vi "viscosity_to_RPM_derate.vi"(8 "base RPM":dbl=350.0, 9 "slope":dbl=-5.2, 10 "viscosity (cP)":dbl) -> (3 "output_RPM":i32)   [LabVIEW 2019]
panel:
  out "output_base_RPM":dbl=380.0
  in  "min_RPM":i32=30
  out "desired_RPM":i32
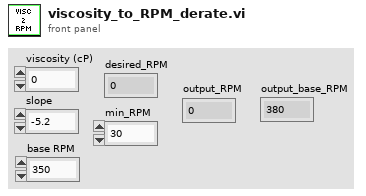
[diagram p1: front panel]
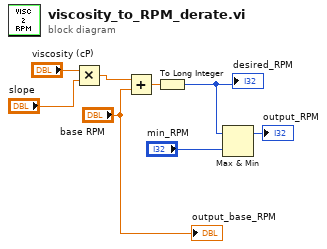
[diagram p0: block diagram]
diagram:
  n1 = Multiply(x="viscosity (cP)", y="slope") -> (x*y=w6:dbl)
  n2 = Add(x=w6, y="base RPM") -> (x+y=w4:dbl)
  n3 = To Long Integer(number=w4) -> (32bit integer=w3:i32)
  "desired_RPM" <- w3
  n4 = Max & Min(x=w3, y="min_RPM") -> (max(x,y)=→"output_RPM":i32)  [unwired: 1 out]
  "output_base_RPM" <- "base RPM"
